vi "ARGB To RGBA.vi"(10 "Depth":i32, 11 "ARGB":u8[](array[numeric])) -> (3 "RGBA":u8[](array[numeric]))   [LabVIEW 2020, in "G-Image.lvlib"]
doc: "Convert the image memory layout from ARGB to RGBA. Applies to 32-bit images only."
uses:
  G-Image.lvlib
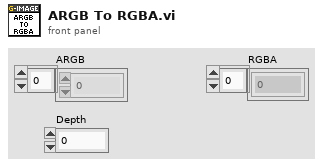
[diagram p1: front panel]
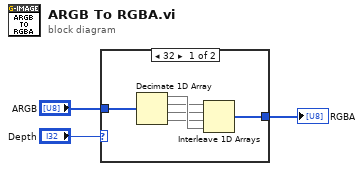
[diagram p0: block diagram]
diagram:
  n1 = case shown="32" "Depth" {
    tunnel: "ARGB" -> [w9 w10]
    tunnel: [w8 w10] -> w1
    frame 32 {
      n2 = Decimate 1D Array(w9) -> (w7:u8[], w6:u8[], w5:u8[], w4:u8[])
      n3 = Interleave 1D Arrays(w6, w5, w4, w7) -> (w8:u8[])
    }
    frame Default {
      # "1, 4, 8, 24"
    }
  }
  "RGBA" <- w1
